vi "TEST - Delete Elements from Array.vi"(8 "error in (no error)":errorcluster) -> (0 "error out":errorcluster, 2 "Pass?":bool=TRUE)   [LabVIEW 2020]
doc: "This VI template can be used for the functional testing of VIs; this implementation includes handling for the testing of polymorphic VIs, and the polymorphic elements should be removed if not needed.\n\nCoded by Douglas A. Femec, January 24, 2006.\n\nCopyright (c) 2005-2006 MKS Instruments, Inc.\nAll rights reserved."
uses:
  TEST - Delete Elements from Array - Inputs.ctl
  Polymorphizer+ Data Type.ctl
  TEST - Delete Elements from Array - Outputs.ctl
  source/library/Delete Elements from Array/Delete Elements from 1D Array (EXT).vi
  source/library/Delete Elements from Array/Delete Elements from 1D Array (I64).vi
  source/library/Delete Elements from Array/Delete Elements from 1D Array (U64).vi
  source/library/Delete Elements from Array/Delete Elements from 1D Array (DBL).vi
  source/library/Delete Elements from Array/Delete Elements from 1D Array (SGL).vi
  source/library/Delete Elements from Array/Delete Elements from 1D Array (I32).vi
  source/library/Delete Elements from Array/Delete Elements from 1D Array (I16).vi
  source/library/Delete Elements from Array/Delete Elements from 1D Array (I8).vi
  source/library/Delete Elements from Array/Delete Elements from 1D Array (LVObject).vi
  source/library/Delete Elements from Array/Delete Elements from 1D Array (U32).vi
  source/library/Delete Elements from Array/Delete Elements from 1D Array (U16).vi
  source/library/Delete Elements from Array/Delete Elements from 1D Array (U8).vi
  source/library/Delete Elements from Array/Delete Elements from 1D Array (CXT).vi
  source/library/Delete Elements from Array/Delete Elements from 1D Array (CDB).vi
  source/library/Delete Elements from Array/Delete Elements from 1D Array (CSG).vi
  source/library/Delete Elements from Array/Delete Elements from 1D Array (Boolean).vi
  source/library/Delete Elements from Array/Delete Elements from 1D Array (String).vi
  source/library/Delete Elements from Array/Delete Elements from 1D Array (Path).vi
  source/library/Delete Elements from Array/Delete Elements from 1D Array (Variant).vi
  TestClass/TestClass.lvclass
panel:
  out "Generated Outputs":T1[][](array[typedef])=[[{"Description"="Expect empty array", "array w/ subset deleted"=[], "deleted elements"=[]}, {"Description"="Expect empty array", "array w/ subset deleted"=[], "deleted elements"=[]}, {"Description"="Expect empty array", "array w/ subset deleted"=[], "deleted elements"=[]}, {"Description"="Expect empty array", "array w/ subset deleted"=[], "deleted elements"=[]}, {"Description"="Expect empty array", "array w/ subset deleted"=[], "deleted elements"=[]}, {"Description"="Expect empty array", "array w/ subset deleted"=[], "deleted elements"=[]}, {"Description"="Expect empty array", "array w/ subset deleted"=[], "deleted elements"=[]}, {"Description"="Expect empty array", "array w/ subset deleted"=[], "deleted elements"=[]}, {"Description"="Expect empty array", "array w/ subset deleted"=[], "deleted elements"=[]}, {"Description"="Expect empty array", "array w/ subset deleted"=[], "deleted elements"=[]}, {"Description"="Expect empty array", "array w/ subset deleted"=[], "deleted elements"=[]}, {"Description"="Expect empty array", "array w/ subset deleted"=[], "deleted elements"=[]}, {"Description"="Expect empty array", "array w/ subset deleted"=[], "deleted elements"=[]}, {"Description"="Expect empty array", "array w/ subset deleted"=[], "deleted elements"=[]}, {"Description"="Expect empty array", "array w/ subset deleted"=[], "deleted elements"=[]}, {"Description"="Expect empty array", "array w/ subset deleted"=[], "deleted elements"=[]}], [{"Description"="Expect no elements deleted", "array w/ subset deleted"=[0.0, 0.0, 0.0, 0.0], "deleted elements"=[]}, {"Description"="Expect no elements deleted", "array w/ subset deleted"=[0.0, 0.0, 0.0, 0.0], "deleted elements"=[]}, {"Description"="Expect no elements deleted", "array w/ subset deleted"=[0.0, 0.0, 0.0, 0.0], "deleted elements"=[]}, {"Description"="Expect no elements deleted", "array w/ subset deleted"=[0.0, 0.0, 0.0, 0.0], "deleted elements"=[]}, {"Description"="Expect no elements deleted", "array w/ subset deleted"=[0.0, 0.0, 0.0, 0.0], "deleted elements"=[]}, {"Description"="Expect no elements deleted", "array w/ subset deleted"=[0.0, 0.0, 0.0, 0.0], "deleted elements"=[]}, {"Description"="Expect no elements deleted", "array w/ subset deleted"=[0.0, 0.0, 0.0, 0.0], "deleted elements"=[]}, {"Description"="Expect no elements deleted", "array w/ subset deleted"=[0.0, 0.0, 0.0, 0.0], "deleted elements"=[]}, {"Description"="Expect no elements deleted", "array w/ subset deleted"=[0.0, 0.0, 0.0, 0.0], "deleted elements"=[]}, {"Description"="Expect no elements deleted", "array w/ subset deleted"=[0.0, 0.0, 0.0, 0.0], "deleted elements"=[]}, {"Description"="Expect no elements deleted", "array w/ subset deleted"=[0.0, 0.0, 0.0, 0.0], "deleted elements"=[]}, {"Description"="Expect no elements deleted", "array w/ subset deleted"=[0.0, 0.0, 0.0, 0.0], "deleted elements"=[]}, {"Description"="Expect no elements deleted", "array w/ subset deleted"=[0.0, 0.0, 0.0, 0.0], "deleted elements"=[]}, {"Description"="Expect no elements deleted", "array w/ subset deleted"=[0.0, 0.0, 0.0, 0.0], "deleted elements"=[]}, {"Description"="Expect no elements deleted", "array w/ subset deleted"=[0.0, 0.0, 0.0, 0.0], "deleted elements"=[]}, {"Description"="Expect no elements deleted", "array w/ subset deleted"=[0.0, 0.0, 0.0, 0.0], "deleted elements"=[]}], [{"Description"="Expect some elements deleted", "array w/ subset deleted"=[3.0, 7.0], "deleted elements"=[1.0, 5.0]}, {"Description"="Expect some elements deleted", "array w/ subset deleted"=[3.0, 7.0], "deleted elements"=[1.0, 5.0]}, {"Description"="Expect some elements deleted", "array w/ subset deleted"=[3.0, 7.0], "deleted elements"=[1.0, 5.0]}, {"Description"="Expect some elements deleted", "array w/ subset deleted"=[3.0, 7.0], "deleted elements"=[1.0, 5.0]}, {"Description"="Expect some elements deleted", "array w/ subset deleted"=[3.0, 7.0], "deleted elements"=[1.0, 5.0]}, {"Description"="Expect some elements deleted", "array w/ subset deleted"=[3.0, 7.0], "deleted elements"=[1.0, 5.0]}, {"Description"="Expect some elements deleted", "array w/ subset deleted"=[3.0, 7.0], "deleted elements"=[1.0, 5.0]}, {"Description"="Expect some elements deleted", "array w/ subset deleted"=[3.0, 7.0], "deleted elements"=[1.0, 5.0]}, {"Description"="Expect some elements deleted", "array w/ subset deleted"=[3.0, 7.0], "deleted elements"=[1.0, 5.0]}, {"Description"="Expect some elements deleted", "array w/ subset deleted"=[3.0, 7.0], "deleted elements"=[1.0, 5.0]}, {"Description"="Expect some elements deleted", "array w/ subset deleted"=[3.0, 7.0], "deleted elements"=[1.0, 5.0]}, {"Description"="Expect some elements deleted", "array w/ subset deleted"=[3.0, 7.0], "deleted elements"=[1.0, 5.0]}, {"Description"="Expect some elements deleted", "array w/ subset deleted"=[3.0, 7.0], "deleted elements"=[1.0, 5.0]}, {"Description"="Expect some elements deleted", "array w/ subset deleted"=[3.0, 7.0], "deleted elements"=[1.0, 5.0]}, {"Description"="Expect some elements deleted", "array w/ subset deleted"=[3.0, 7.0], "deleted elements"=[1.0, 5.0]}, {"Description"="", "array w/ subset deleted"=[], "deleted elements"=[]}], [{"Description"="Deleted Elements", "array w/ subset deleted"=[], "deleted elements"=[6.0, 2.0, 4.0, 0.0]}, {"Description"="Deleted Elements", "array w/ subset deleted"=[], "deleted elements"=[6.0, 2.0, 4.0, 0.0]}, {"Description"="Deleted Elements", "array w/ subset deleted"=[], "deleted elements"=[6.0, 2.0, 4.0, 0.0]}, {"Description"="Deleted Elements", "array w/ subset deleted"=[], "deleted elements"=[6.0, 2.0, 4.0, 0.0]}, {"Description"="Deleted Elements", "array w/ subset deleted"=[], "deleted elements"=[6.0, 2.0, 4.0, 0.0]}, {"Description"="Deleted Elements", "array w/ subset deleted"=[], "deleted elements"=[6.0, 2.0, 4.0, 0.0]}, {"Description"="Deleted Elements", "array w/ subset deleted"=[], "deleted elements"=[6.0, 2.0, 4.0, 0.0]}, {"Description"="Deleted Elements", "array w/ subset deleted"=[], "deleted elements"=[6.0, 2.0, 4.0, 0.0]}, {"Description"="Deleted Elements", "array w/ subset deleted"=[], "deleted elements"=[6.0, 2.0, 4.0, 0.0]}, {"Description"="Deleted Elements", "array w/ subset deleted"=[], "deleted elements"=[6.0, 2.0, 4.0, 0.0]}, {"Description"="Deleted Elements", "array w/ subset deleted"=[], "deleted elements"=[6.0, 2.0, 4.0, 0.0]}, {"Description"="Deleted Elements", "array w/ subset deleted"=[], "deleted elements"=[6.0, 2.0, 4.0, 0.0]}, {"Description"="Deleted Elements", "array w/ subset deleted"=[], "deleted elements"=[6.0, 2.0, 4.0, 0.0]}, {"Description"="Deleted Elements", "array w/ subset deleted"=[], "deleted elements"=[6.0, 2.0, 4.0, 0.0]}, {"Description"="Deleted Elements", "array w/ subset deleted"=[], "deleted elements"=[6.0, 2.0, 4.0, 0.0]}, {"Description"="", "array w/ subset deleted"=[], "deleted elements"=[]}]] {"deleted elements" format="%.2f"; "array w/ subset deleted" format="%.2f"}
  in  "Expected Outputs":T1[](array[typedef])=[{"Description"="Expect empty array", "array w/ subset deleted"=[], "deleted elements"=[]}, {"Description"="Expect no elements deleted", "array w/ subset deleted"=[0.0, 0.0, 0.0, 0.0], "deleted elements"=[]}, {"Description"="Expect some elements deleted", "array w/ subset deleted"=[3.0, 7.0], "deleted elements"=[1.0, 5.0]}, {"Description"="Deleted Elements", "array w/ subset deleted"=[], "deleted elements"=[6.0, 2.0, 4.0, 0.0]}] {"deleted elements" format="%.2f"; "array w/ subset deleted" format="%.2f"}
  in  "Inputs":T2[](array[typedef])=[{"Description"="Empty arrays", "Data Types to Test"=[enum."EXT", enum."DBL", enum."SGL", enum."I32", enum."I16", enum."I8", enum."U32", enum."U16", enum."U8", enum."CXT", enum."CDB", enum."CSG", enum."Boolean", enum."String", enum."Path", enum."Variant", enum."I64", enum."U64", enum."LabVIEW Object"], "Array"=[], "Indices"=[]}, {"Description"="No elements to delete", "Data Types to Test"=[enum."EXT", enum."DBL", enum."SGL", enum."I32", enum."I16", enum."I8", enum."U32", enum."U16", enum."U8", enum."CXT", enum."CDB", enum."CSG", enum."Boolean", enum."String", enum."Path", enum."Variant", enum."I64", enum."U64", enum."LabVIEW Object"], "Array"=[0.0, 0.0, 0.0, 0.0], "Indices"=[]}, {"Description"="Delete some elements", "Data Types to Test"=[enum."EXT", enum."DBL", enum."SGL", enum."I32", enum."I16", enum."I8", enum."U32", enum."U16", enum."U8", enum."CXT", enum."CDB", enum."CSG", enum."String", enum."Path", enum."Variant", enum."I64", enum."U64", enum."LabVIEW Object"], "Array"=[1.0, 3.0, 5.0, 7.0], "Indices"=[0, 2]}, {"Description"="Delete All Elements", "Data Types to Test"=[enum."EXT", enum."DBL", enum."SGL", enum."I32", enum."I16", enum."I8", enum."U32", enum."U16", enum."U8", enum."CXT", enum."CDB", enum."CSG", enum."String", enum."Path", enum."Variant", enum."I64", enum."U64", enum."LabVIEW Object"], "Array"=[6.0, 4.0, 2.0, 0.0], "Indices"=[0, 2, 1, 3]}] {"Array" format="%.2f"}
  # "Copyright (c) 2005-2006 MKS Instruments, Inc.\nAll rights reserved."
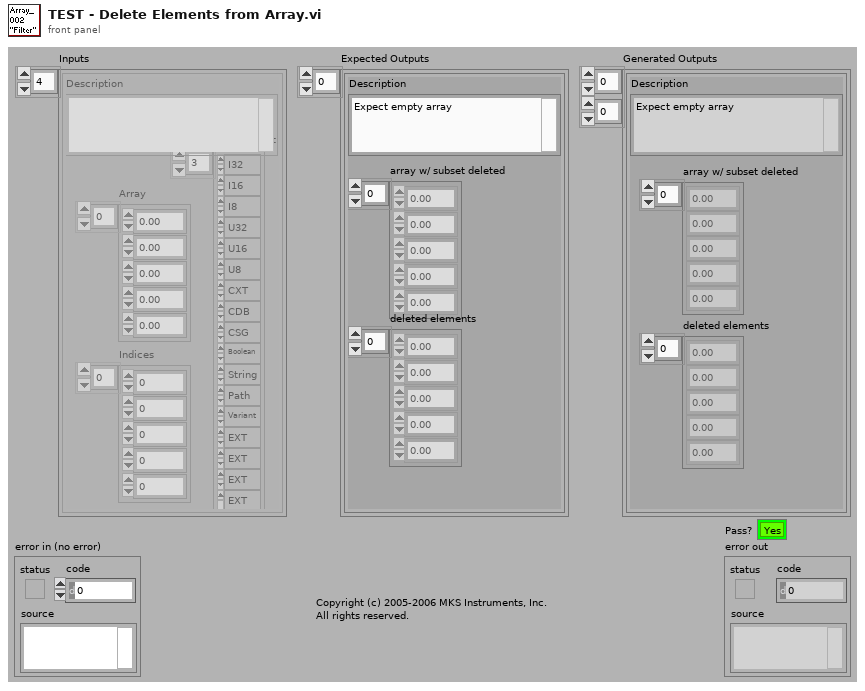
[diagram p1: front panel]
types:
  T1 = typedef "TEST - Delete Elements from Array - Outputs.ctl" = cluster{"Description":string, "array w/ subset deleted":sgl[], "deleted elements":sgl[]}
  T2 = typedef "TEST - Delete Elements from Array - Inputs.ctl" = cluster{"Description":string, "Data Types to Test":T3[], "Array":sgl[], "Indices":i32[]}
  T3 = typedef "Polymorphizer+ Data Type.ctl" = enum16{"EXT", "DBL", "SGL", "I32", "I16", "I8", "U32", "U16", "U8", "CXT", "CDB", "CSG", "Boolean", "String", "Path", "Variant", "CTL-REF", "GEN-REF", "GObj-REF", "VI-REF", "ENUM", "ERR", "FILE-REF", "MENU-REF", "MENU-RING", "PICT-RING", "TXT&PICT-RING", "TXT-RING", "I64", "U64", "LabVIEW Object"}
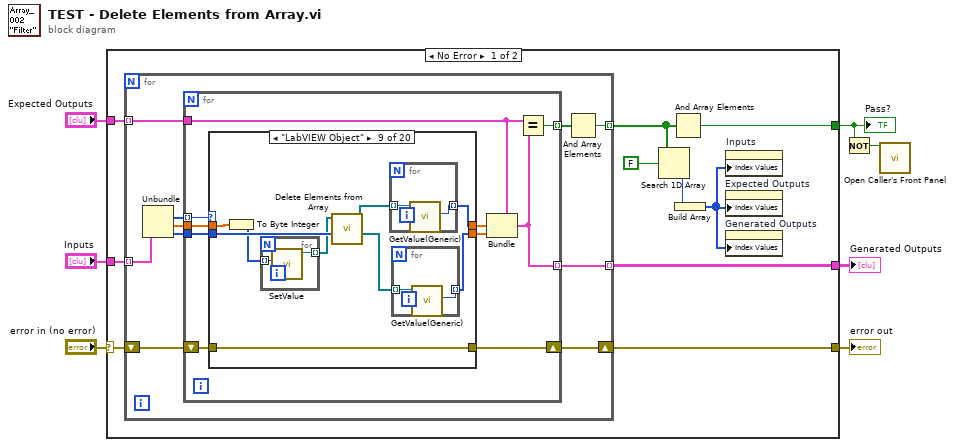
[diagram p0: block diagram]
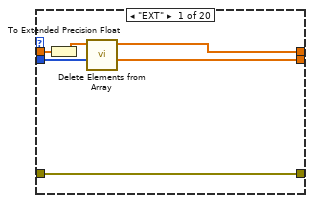
[diagram p2: hidden frame]
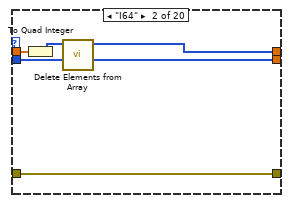
[diagram p3: hidden frame]
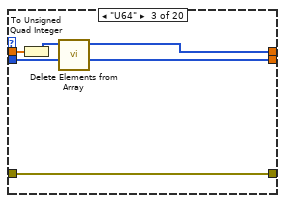
[diagram p4: hidden frame]
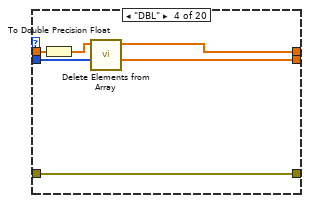
[diagram p5: hidden frame]
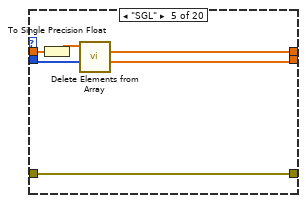
[diagram p6: hidden frame]
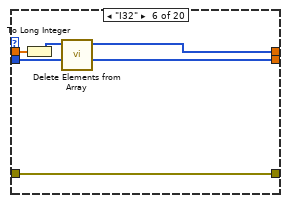
[diagram p7: hidden frame]
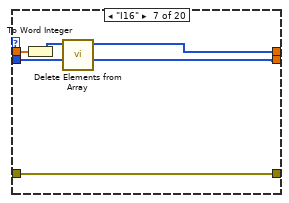
[diagram p8: hidden frame]
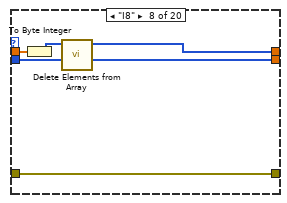
[diagram p9: hidden frame]
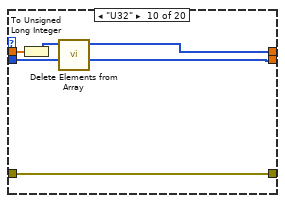
[diagram p10: hidden frame]
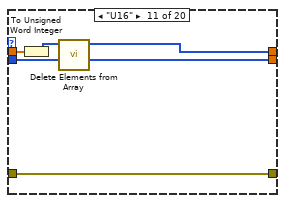
[diagram p11: hidden frame]
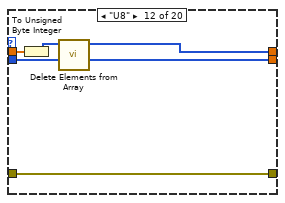
[diagram p12: hidden frame]
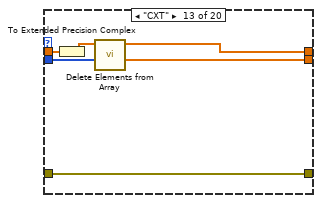
[diagram p13: hidden frame]
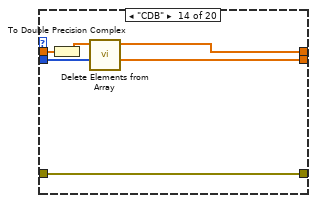
[diagram p14: hidden frame]
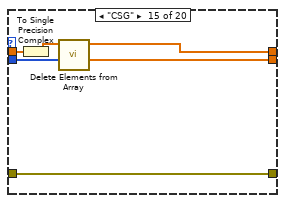
[diagram p15: hidden frame]
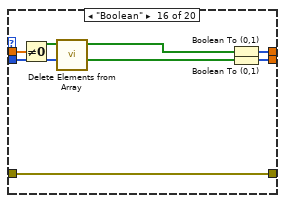
[diagram p16: hidden frame]
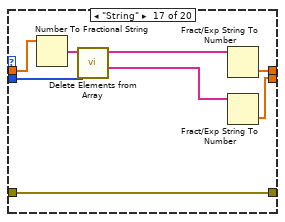
[diagram p17: hidden frame]
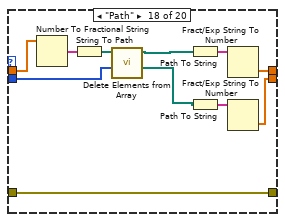
[diagram p18: hidden frame]
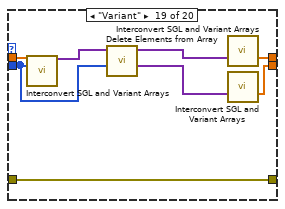
[diagram p19: hidden frame]
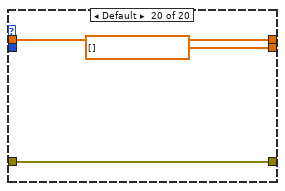
[diagram p20: hidden frame]
diagram:
  n1 = case shown="No Error" "error in (no error)" {
    selector: "error in (no error)" -> [w16 w175]
    tunnel: [w17 w175] -> w6
    tunnel: "Expected Outputs" -> [w14 _]
    tunnel: "Inputs" -> [w15 _]
    tunnel: [w13 _] -> w3
    tunnel: [w12 _] -> w2
    frame No Error {
      n2 = for {
        shift-right: [w22] -> w17
        shift-left: w16 -> [w23]
        tunnel: w15 -> [w24] mode=indexing
        tunnel: w14 -> [w27] mode=indexing
        tunnel: [w26] -> w13 mode=indexing
        tunnel: [w21] -> w11 mode=indexing
        n3 = Unbundle(w24) -> ("Data Types to Test"=w20:T3[], "Array"=w18:sgl[], "Indices"=w19:i32[])  [unwired: 1 out]
        n4 = for {
          tunnel: w27 -> [w37]
          tunnel: [w35] -> w26 mode=indexing
          tunnel: [w36] -> w25 mode=indexing
          shift-right: [w30] -> w22
          shift-left: w23 -> [w31]
          tunnel: w20 -> [w32] mode=indexing
          tunnel: w18 -> [w34]
          tunnel: w19 -> [w33]
          n5 = case shown="\"LabVIEW Object\"" w32 {
            tunnel: w34 -> [w43 w49 w55 w61 w67 w73 w79 w85 w94 w106 w112 w118 w124 w130 w136 w144 w152 w162 w170 w173]
            tunnel: [w39 w45 w51 w57 w63 w69 w74 w80 w87 w101 w107 w113 w119 w125 w131 w143 w151 w161 w169 w173] -> w29
            tunnel: w33 -> [w40 w46 w52 w59 w64 w71 w77 w83 w92 w104 w110 w116 w122 w128 w134 w140 w149 w158 w168 _]
            tunnel: w31 -> [w42 w48 w54 w60 w66 w72 w78 w84 w93 w105 w111 w117 w123 w129 w135 w142 w150 w159 w171 w174]
            tunnel: [w42 w48 w54 w60 w66 w72 w78 w84 w93 w105 w111 w117 w123 w129 w135 w142 w150 w159 w171 w174] -> w30
            tunnel: [w38 w44 w50 w56 w62 w68 w75 w81 w89 w102 w108 w114 w120 w126 w132 w138 w145 w153 w165 cxt[] []] -> w28
            frame "EXT" {
              n6 = To Extended Precision Float(1:w43) -> (0:w41:ext[])
              n7 = call-poly "Delete Elements from Array.vi"("indices"=w40, "array"=w41) -> ("deleted elements"=w38:ext[], "array w/ subset deleted"=w39:ext[])  [unwired: 8 in]
            }
            frame "I64" {
              n8 = To Quad Integer(1:w49) -> (0:w47:i64[])
              n9 = call-poly "Delete Elements from Array.vi"("indices"=w46, "array"=w47) -> ("deleted elements"=w44:i64[], "array w/ subset deleted"=w45:i64[])  [unwired: 8 in]
            }
            frame "U64" {
              n10 = To Unsigned Quad Integer(1:w55) -> (0:w53:u64[])
              n11 = call-poly "Delete Elements from Array.vi"("indices"=w52, "array"=w53) -> ("deleted elements"=w50:u32[], "array w/ subset deleted"=w51:u64[])  [unwired: 8 in]
            }
            frame "DBL" {
              n12 = To Double Precision Float(number=w61) -> (double precision float=w58:dbl[])
              n13 = call-poly "Delete Elements from Array.vi"("indices"=w59, "array"=w58) -> ("deleted elements"=w56:dbl[], "array w/ subset deleted"=w57:dbl[])  [unwired: 8 in]
            }
            frame "SGL" {
              n14 = To Single Precision Float(number=w67) -> (single precision float=w65:sgl[])
              n15 = call-poly "Delete Elements from Array.vi"("indices"=w64, "array"=w65) -> ("deleted elements"=w62:sgl[], "array w/ subset deleted"=w63:sgl[])  [unwired: 8 in]
            }
            frame "I32" {
              n16 = To Long Integer(number=w73) -> (32bit integer=w70:i32[])
              n17 = call-poly "Delete Elements from Array.vi"("indices"=w71, "array"=w70) -> ("deleted elements"=w68:i32[], "array w/ subset deleted"=w69:i32[])  [unwired: 8 in]
            }
            frame "I16" {
              n18 = To Word Integer(number=w79) -> (16bit integer=w76:i16[])
              n19 = call-poly "Delete Elements from Array.vi"("indices"=w77, "array"=w76) -> ("deleted elements"=w75:i16[], "array w/ subset deleted"=w74:i16[])  [unwired: 8 in]
            }
            frame "I8" {
              n20 = To Byte Integer(number=w85) -> (8bit integer=w82:i8[])
              n21 = call-poly "Delete Elements from Array.vi"("indices"=w83, "array"=w82) -> ("deleted elements"=w81:i8[], "array w/ subset deleted"=w80:i8[])  [unwired: 8 in]
            }
            frame "LabVIEW Object" {
              n22 = To Byte Integer(number=w94) -> (8bit integer=w91:i8[])
              n23 = for {
                tunnel: w91 -> [w100] mode=indexing
                tunnel: [w99] -> w90 mode=indexing
                n24 = call "SetValue.vi"("Value"=w100) -> ("TestClass out"=w99:refnum<class "TestClass.lvclass">)  [unwired: 9 in, 1 out]
              }
              n25 = call-poly "Delete Elements from Array.vi"("indices"=w92, "array"=w90) -> ("deleted elements"=w88:refnum<class>[], "array w/ subset deleted"=w86:refnum<class>[])  [unwired: 8 in]
              n26 = for {
                tunnel: w86 -> [w96] mode=indexing
                tunnel: [w95] -> w87 mode=indexing
                n27 = call "GetValue(Generic).vi"("TestClass in"=w96) -> ("Value"=w95:i32)  [unwired: 8 in, 2 out]
              }
              n28 = for {
                tunnel: w88 -> [w98] mode=indexing
                tunnel: [w97] -> w89 mode=indexing
                n29 = call "GetValue(Generic).vi"("TestClass in"=w98) -> ("Value"=w97:i32)  [unwired: 8 in, 2 out]
              }
            }
            frame "U32" {
              n30 = To Unsigned Long Integer(number=w106) -> (unsigned 32bit integer=w103:u32[])
              n31 = call-poly "Delete Elements from Array.vi"("indices"=w104, "array"=w103) -> ("deleted elements"=w102:u32[], "array w/ subset deleted"=w101:u32[])  [unwired: 8 in]
            }
            frame "U16" {
              n32 = To Unsigned Word Integer(number=w112) -> (unsigned 16bit integer=w109:u16[])
              n33 = call-poly "Delete Elements from Array.vi"("indices"=w110, "array"=w109) -> ("deleted elements"=w108:u16[], "array w/ subset deleted"=w107:u16[])  [unwired: 8 in]
            }
            frame "U8" {
              n34 = To Unsigned Byte Integer(number=w118) -> (unsigned 8bit integer=w115:u8[])
              n35 = call-poly "Delete Elements from Array.vi"("indices"=w116, "array"=w115) -> ("deleted elements"=w114:u8[], "array w/ subset deleted"=w113:u8[])  [unwired: 8 in]
            }
            frame "CXT" {
              n36 = To Extended Precision Complex(1:w124) -> (0:w121:cxt[])
              n37 = call-poly "Delete Elements from Array.vi"("indices"=w122, "array"=w121) -> ("deleted elements"=w120:cxt[], "array w/ subset deleted"=w119:cxt[])  [unwired: 8 in]
            }
            frame "CDB" {
              n38 = To Double Precision Complex(1:w130) -> (0:w127:cdb[])
              n39 = call-poly "Delete Elements from Array.vi"("indices"=w128, "array"=w127) -> ("deleted elements"=w126:cdb[], "array w/ subset deleted"=w125:cdb[])  [unwired: 8 in]
            }
            frame "CSG" {
              n40 = To Single Precision Complex(1:w136) -> (0:w133:csg[])
              n41 = call-poly "Delete Elements from Array.vi"("indices"=w134, "array"=w133) -> ("deleted elements"=w132:csg[], "array w/ subset deleted"=w131:csg[])  [unwired: 8 in]
            }
            frame "Boolean" {
              n42 = Not Equal To 0?(x=w144) -> (x != 0?=w141:bool[])
              n43 = call-poly "Delete Elements from Array.vi"("indices"=w140, "array"=w141) -> ("deleted elements"=w137:bool[], "array w/ subset deleted"=w139:bool[])  [unwired: 8 in]
              n44 = Boolean To (0,1)(Boolean=w139) -> (0, 1=w143:i16[])
              n45 = Boolean To (0,1)(Boolean=w137) -> (0, 1=w138:i16[])
            }
            frame "String" {
              n46 = Number To Fractional String(number=w152) -> (F-format string=w148:string[])  [unwired: 3 in]
              n47 = call-poly "Delete Elements from Array.vi"("indices"=w149, "array"=w148) -> ("deleted elements"=w146:string[], "array w/ subset deleted"=w147:string[])  [unwired: 8 in]
              n48 = Fract/Exp String To Number(string=w147) -> (number=w151:dbl[])  [unwired: 3 in, 1 out]
              n49 = Fract/Exp String To Number(string=w146) -> (number=w145:dbl[])  [unwired: 3 in, 1 out]
            }
            frame "Path" {
              n50 = Number To Fractional String(number=w162) -> (F-format string=w163:string[])  [unwired: 3 in]
              n51 = String To Path(string=w163) -> (path=w157:path[])
              n52 = call-poly "Delete Elements from Array.vi"("indices"=w158, "array"=w157) -> ("deleted elements"=w154:path[], "array w/ subset deleted"=w156:path[])  [unwired: 8 in]
              n53 = Path To String(path=w156) -> (string=w160:string[])
              n54 = Path To String(path=w154) -> (string=w155:string[])
              n55 = Fract/Exp String To Number(string=w160) -> (number=w161:dbl[])  [unwired: 3 in, 1 out]
              n56 = Fract/Exp String To Number(string=w155) -> (number=w153:dbl[])  [unwired: 3 in, 1 out]
            }
            frame "Variant" {
              n57 = call "Interconvert SGL and Variant Arrays.vi"("SGL 1D Array In"=w170, "SGL 1D Array 2 In"=w168) -> ("Variant 1D Array Out"=w167:variant[])  [unwired: 9 in, 4 out]
              n58 = call-poly "Delete Elements from Array.vi"("indices"=w168, "array"=w167) -> ("deleted elements"=w164:variant[], "array w/ subset deleted"=w166:variant[])  [unwired: 8 in]
              n59 = call "Interconvert SGL and Variant Arrays.vi"("Variant 1D Array In"=w166) -> ("SGL 1D Array Out"=w169:sgl[])  [unwired: 10 in, 4 out]
              n60 = call "Interconvert SGL and Variant Arrays.vi"("Variant 1D Array In"=w164) -> ("SGL 1D Array Out"=w165:sgl[])  [unwired: 10 in, 4 out]
            }
            frame Default {
            }
          }
          n61 = Bundle(cluster=w37, "array w/ subset deleted"=w29, "deleted elements"=w28) -> (w35:T1)  [unwired: 1 in]
          n62 = Equal?(x=w37, y=w35) -> (x = y?=w36:bool)
        }
        n63 = And Array Elements(Boolean array=w25) -> (logical AND=w21:bool)
      }
      n64 = Search 1D Array(1D array=w11, element=FALSE) -> (index of element=w9:i32)  [unwired: 1 in]
      n65 = And Array Elements(Boolean array=w11) -> (logical AND=w12:bool)
      n66 = Build Array(w9) -> (w8:i32[])
      n67 = property on="Inputs" class="Arr (strict)"("Index Values"=w8) -> ()  [unwired: 2 in, 2 out]
      n68 = property on="Expected Outputs" class="Arr (strict)"("Index Values"=w8) -> ()  [unwired: 2 in, 2 out]
      n69 = property on="Generated Outputs" class="Arr (strict)"("Index Values"=w8) -> ()  [unwired: 2 in, 2 out]
    }
    frame Error {
    }
  }
  "error out" <- w6
  "Pass?" <- w2
  "Generated Outputs" <- w3
  n70 = Not(x=w2) -> (.not. x?=w1:bool)
  n71 = call "Open Caller's Front Panel.vi"("Open?"=w1) -> ()  [unwired: 14 in, 1 out]
